vi "MessageName.vi"() -> (2 "MessageName":string)   [LabVIEW 2020, in "TcpReply.lvlib"]
uses:
  TcpReply.lvlib
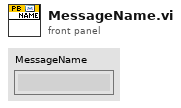
[diagram p1: front panel]
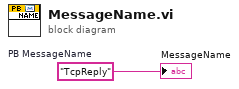
[diagram p0: block diagram]
diagram:
  w1 = "TcpReply"  # PB MessageName
  "MessageName" <- w1
